vi "RH Correction Via PWM.vi"(1 "Fan Flowrate, System Volume":dbl[](array[numeric]), 2 "Max Humidity (%)":u8, 3 "System RH":u8, 4 "System Temp (C)":u8, 5 "Environment Temp (C)":u8, 6 "Environment RH":u8) -> (0 "Time to Run PWM":dbl)   [LabVIEW 2020]
panel:
  in  "stop":bool
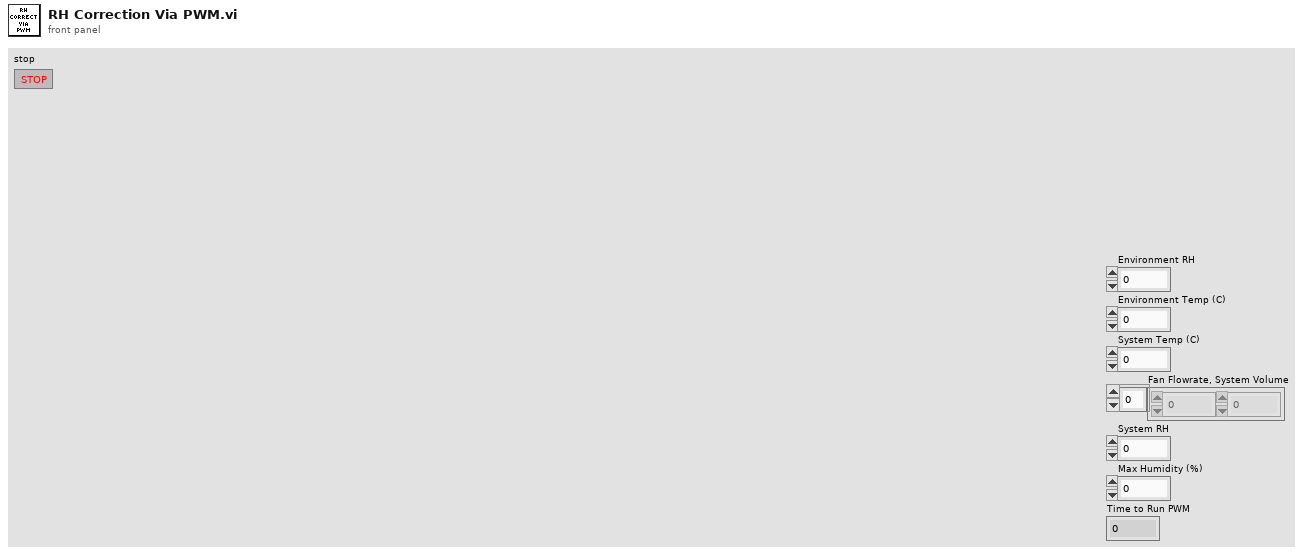
[diagram p1: front panel]
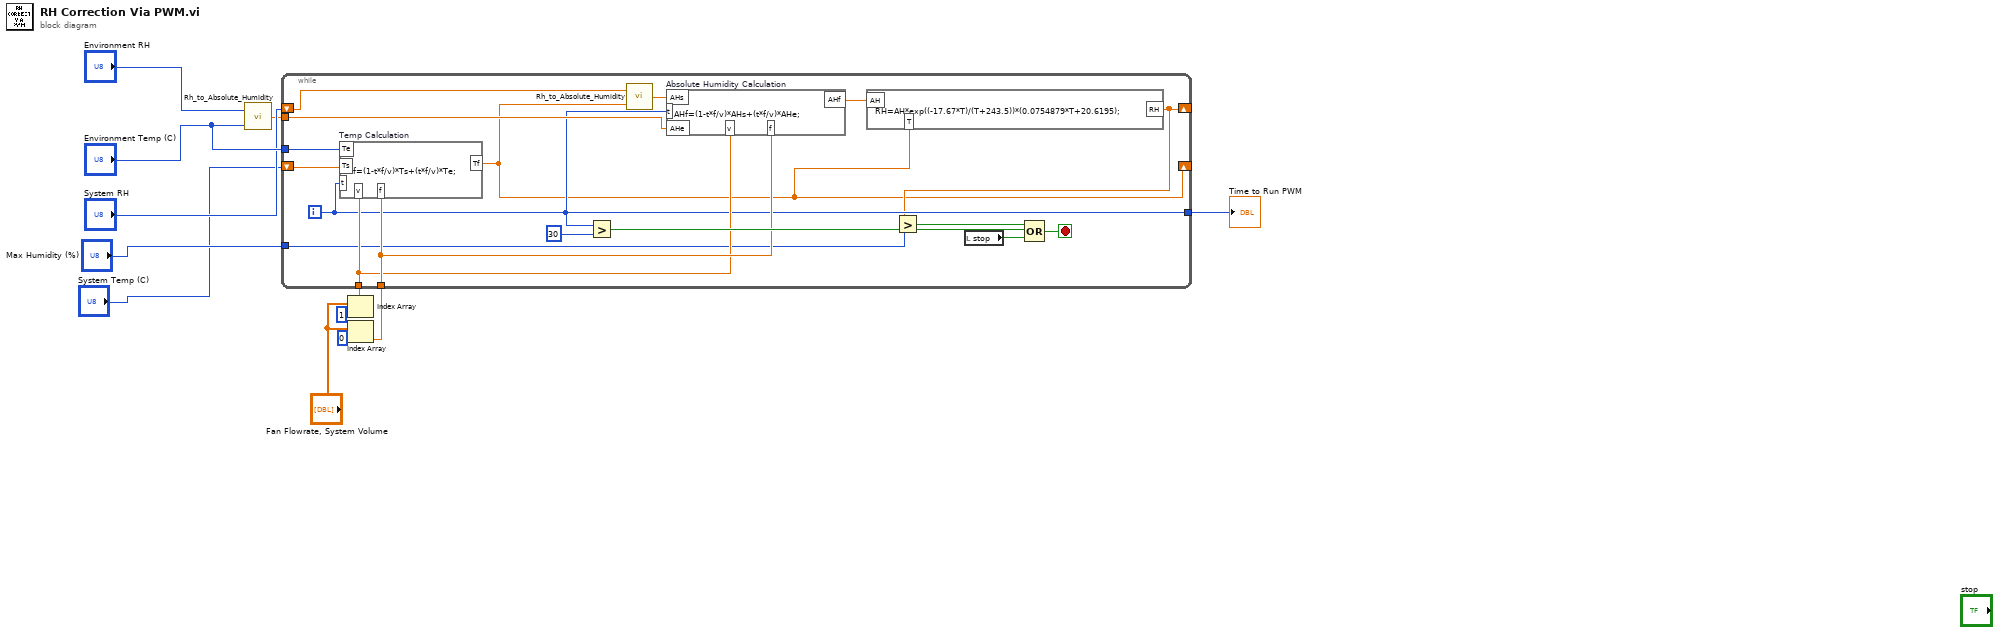
[diagram p0: block diagram]
diagram:
  n1 = call "Rh_to_Absolute_Humidity.vi"("Temperature (F)"="Environment Temp (C)", "Relative Humidity"="Environment RH") -> ("Absolute Humidity"=w5:dbl)
  n2 = Index Array(array="Fan Flowrate, System Volume", index=1) -> (element=w1:dbl)
  n3 = Index Array(array="Fan Flowrate, System Volume", index=0) -> (element=w2:dbl)
  n4 = while {
    tunnel: "Environment Temp (C)" -> [w24]
    tunnel: w1 -> [w21]
    tunnel: w2 -> [w22]
    shift-right: [w13] -> _
    shift-left: "System Temp (C)" -> [w29]
    tunnel: w5 -> [w20]
    shift-right: [w17] -> _
    shift-left: "System RH" -> [w25]
    tunnel: [w19] -> w6
    tunnel: "Max Humidity (%)" -> [w16]
    i -> [w19]
    stop <- w28 stop-if-true
    n5 = formula code="Tf=(1-t*f/v)*Ts+(t*f/v)*Te;" "Temp Calculation"("Te"=w24, "Ts"=w29, "t"=w19, "v"=w21, "f"=w22) -> ("Tf"=w13:dbl)
    n6 = Greater?(x=w19, y=30) -> (0:w27:bool)
    n7 = call "Rh_to_Absolute_Humidity.vi"("Temperature (F)"=w13, "Relative Humidity"=w25) -> ("Absolute Humidity"=w23:dbl)
    n8 = formula code="AHf=(1-t*f/v)*AHs+(t*f/v)*AHe;" "Absolute Humidity Calculation"("AHs"=w23, "AHe"=w20, "v"=w21, "f"=w22, "t"=w19) -> ("AHf"=w18:dbl)
    n9 = formula code="RH=AH*exp((-17.67*T)/(T+243.5))*(0.0754879*T+20.6195);"("AH"=w18, "T"=w13) -> ("RH"=w17:dbl)
    n10 = Greater?(x=w17, y=w16) -> (0:w15:bool)
    n11 = local read "stop"() -> (w14:bool)
    n12 = Compound Arithmetic op=OR(w15, w27, w14) -> (w28:bool)
  }
  "Time to Run PWM" <- w6
